vi "3 Tap 14-Bit.vi"() -> (0 "Pixels":T1)   [LabVIEW 2013]
uses:
  <vilib>/rvi/eio/common/nirviEmuTemplateMethod_errors.vi
  <vilib>/eio/EIONode/EIONode.xnode
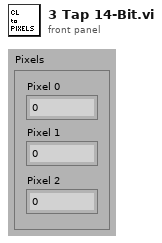
[diagram p1: front panel]
types:
  T1 = cluster{"Pixel 0":u16, "Pixel 1":u16, "Pixel 2":u16}
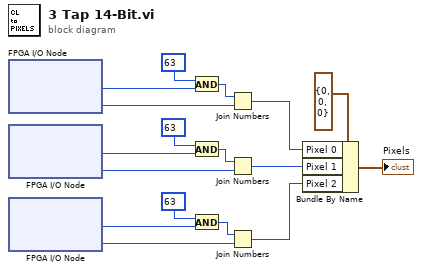
[diagram p0: block diagram]
diagram:
  n1 = xnode "FPGA I/O Node"() -> ("CL Port B"=w8:u8, "CL Port A"=w7:u8)  [unwired: 2 in, 2 out]
  n2 = xnode "FPGA I/O Node"() -> ("CL Port E"=w5:u8, "CL Port D"=w4:u8)  [unwired: 2 in, 2 out]
  n3 = xnode "FPGA I/O Node"() -> ("CL Port F"=w9:u8, "CL Port C"=w6:u8)  [unwired: 2 in, 2 out]
  n4 = And(x=u8 63 ("hi"), y=w8) -> (x .and. y?=w14:u8)
  n5 = And(x=u8 63 ("hi"), y=w5) -> (x .and. y?=w10:u8)
  n6 = And(x=u8 63 ("hi"), y=w9) -> (x .and. y?=w12:u8)
  n7 = Join Numbers(hi=w14, lo=w7) -> ((hi.lo)=w3:u16)
  n8 = Join Numbers(hi=w10, lo=w4) -> ((hi.lo)=w2:u16)
  n9 = Join Numbers(hi=w12, lo=w6) -> ((hi.lo)=w1:u16)
  n10 = Bundle By Name(cluster=T1 {"Pixel 0"=0, "Pixel 1"=0, "Pixel 2"=0} ("PixelData"), "Pixel 0"=w3, "Pixel 1"=w2, "Pixel 2"=w1) -> (→"Pixels":T1)
